vi "vision3.vi"(0 "Red BCG Values (Brightness 1)":T1={"Brightness"=1.0, "Contrast"=89.0, "Gamma"=10.0}, 1 "Green BCG Values (Brightness 1)":T1={"Brightness"=1.0, "Contrast"=89.0, "Gamma"=10.0}, 2 "Blue BCG Values (Brightness 1)":T1={"Brightness"=1.0, "Contrast"=89.0, "Gamma"=10.0}, 3 "Color Mode (Color Threshold 1)":u16(ring) items=["RGB", "HSL", "HSV", "HSI"], 4 "Red or Hue Range (Color Threshold 1)":cluster{"Lower value":i32, "Upper value":i32}={"Lower value"=239, "Upper value"=255}, 5 "Green or Sat Range (Color Threshold 1)":cluster{"Lower value":i32, "Upper value":i32}, 6 "Blue or Luma or Val or Inten Range (Color Threshold 1)":cluster{"Lower value":i32, "Upper value":i32}, 7 "error in":errorcluster) -> (20 "Centroid (Centroid 1)":cluster{"X Centroid":sgl, "Y Centroid":sgl} {"Y Centroid" format="%.2f"; "X Centroid" format="%.2f"}, 21 "Calibrated Centroid (Centroid 1)":cluster{"X Centroid":sgl, "Y Centroid":sgl} {"Y Centroid" format="%.2f"; "X Centroid" format="%.2f"}, 27 "error out":errorcluster)   [LabVIEW 2016]
uses:
  <vilib>/vision/driver/NI_Vision_Acquisition_Software.lvlib
  <vilib>/vision/NI_Vision_Development_Module.lvlib
panel:
  out "Image Out":T2(plugin-control)
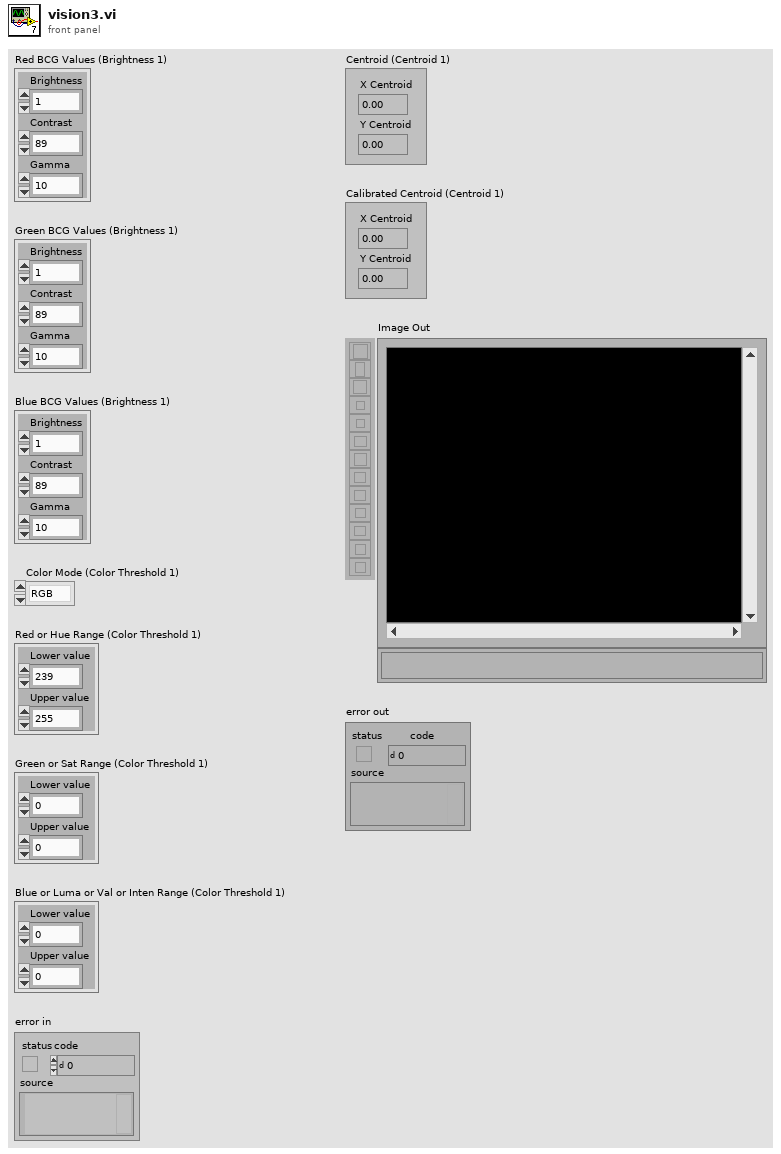
[diagram p1: front panel]
types:
  T1 = cluster{"Brightness":sgl, "Contrast":sgl, "Gamma":sgl}
  T2 = typedef "IMAQ Image.ctl" = refnum<image>
  T3 = typedef "IMAQdx.ctl" = refnum<k21>
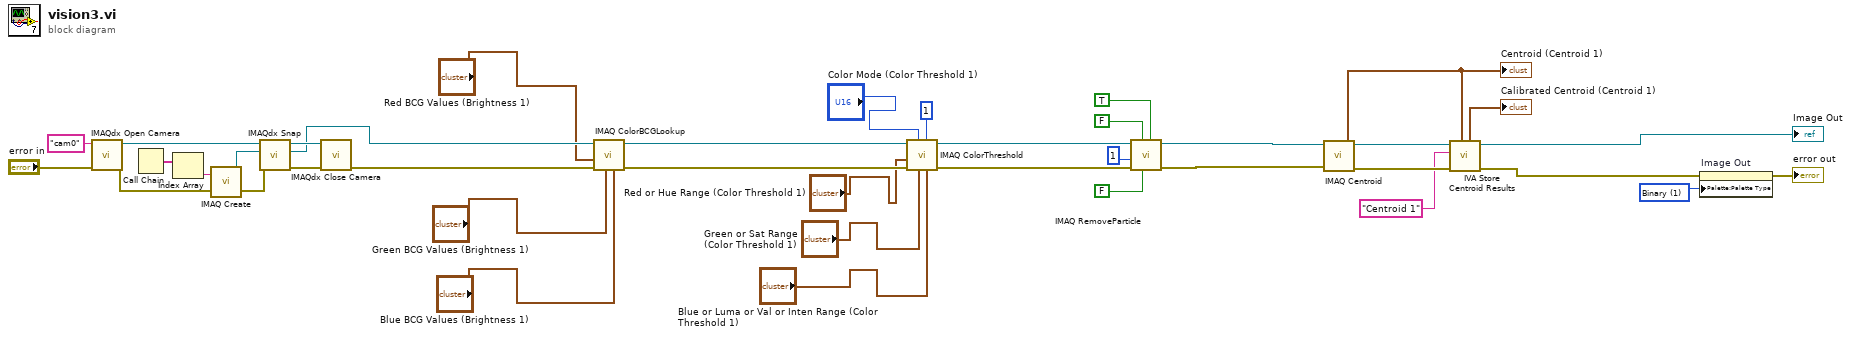
[diagram p0: block diagram]
diagram:
  w1 = u32 1 items=["Grayscale", "Binary", "Gradient", "Rainbow", "Temperature", "User Defined", "Binary 16 Bit", "Gradient 16 Bit", "Rainbow 16 Bit", "Temperature 16 Bit", "User Defined 16 Bit"] ("Palette Type")
  n1 = call <vilib>:"IMAQdx Open Camera.vi"("error in"="error in", "Session In"="cam0" ("Interface Name")) -> ("error out"=w37:errorcluster, "Session Out"=w31:T3)  [unwired: 1 in, 7 out]
  n2 = Call Chain() -> (call chain=w29:string[])
  n3 = Index Array(array=w29) -> (element=w28:string)  [unwired: 1 in]
  n4 = call "IMAQ Create"("Image Name"=w28, "error in (no error)"=w37) -> ("New Image"=w33:T2, "error out"=w32:errorcluster)  [unwired: 2 in, 1 out]
  n5 = call <vilib>:"IMAQdx Snap.vi"("error in"=w32, "Image In"=w33, "Session In"=w31) -> ("error out"=w35:errorcluster, "Image Out"=w27:T2, "Session Out"=w36:T3)  [unwired: 6 out]
  n6 = call <vilib>:"IMAQdx Close Camera.vi"("error in"=w35, "Session In"=w36) -> ("error out"=w34:errorcluster)  [unwired: 9 out]
  n7 = call "IMAQ ColorBCGLookup"("Blue BCG Values"="Blue BCG Values (Brightness 1)", "Green BCG Values"="Green BCG Values (Brightness 1)", "error in (no error)"=w34, "Red BCG Values"="Red BCG Values (Brightness 1)", "Image Src"=w27) -> ("error out"=w26:errorcluster, "Image Dst Out"=w17:T2)  [unwired: 2 in, 3 out]
  n8 = call "IMAQ ColorThreshold"("Blue or Luma or Val or Inten Range"="Blue or Luma or Val or Inten Range (Color Threshold 1)", "Replace Value"=1, "Green or Sat Range"="Green or Sat Range (Color Threshold 1)", "Color Mode"="Color Mode (Color Threshold 1)", "error in (no error)"=w26, "Red or Hue Range"="Red or Hue Range (Color Threshold 1)", "Image Src"=w17) -> ("error out"=w16:errorcluster, "Image Dst Out"=w11:T2)  [unwired: 1 in, 2 out]
  n9 = call "IMAQ RemoveParticle"("Connectivity 4/8 (8)"=TRUE, "Low Pass/High Pass (Low)"=FALSE, "Square/Hexa (Square)"=FALSE, "error in (no error)"=w16, "Number of Erosion"=1, "Image Src"=w11) -> ("error out"=w10:errorcluster, "Image Dst Out"=w7:T2)  [unwired: 1 in, 3 out]
  n10 = call "IMAQ Centroid"("error in (no error)"=w10, "Image"=w7) -> ("error out"=w9:errorcluster, "Centroid"=w5:cluster{"X Centroid":sgl, "Y Centroid":sgl})  [unwired: 1 in, 1 out]
  "Centroid (Centroid 1)" <- w5
  n11 = call <vilib>:"IVA Store Centroid Results.vi"("Centroid in"=w5, "error in (no error)"=w9, "Step Name"="Centroid 1", "Image in"=w7) -> ("error out"=w8:errorcluster, "Image dup"=→"Image Out":T2, "Calibrated Centroid"=→"Calibrated Centroid (Centroid 1)":cluster{"X":sgl, "Y":sgl})  [unwired: 5 out]
  n12 = property on="Image Out" class="ImageControl"(error in=w8, "Palette:Palette Type"=w1) -> (error out=→"error out":errorcluster)  [unwired: 1 in, 1 out]
